vi "Configure AI Filter.vi"(0 "VISA resource name":refnum<visa-resource-name>, 5 "Channel No. (1)":i32=1 min=1 max=6932, 9 "Filter Coefficient(3)":i32=3 min=3 max=300, 11 "error in (no error)":errorcluster) -> (4 "VISA resource name out":refnum<visa-resource-name>, 8 "Channel No.":i32, 15 "error out":errorcluster)   [LabVIEW 2020, in "Yokogawa GX Series.lvlib"]
doc: "Sets the first-order lag filter of the high-speed AI channel.\n\nCommand: SFilter."
uses:
  <instrlib>/Yokogawa GX Series/Yokogawa GX Series.lvlib
panel:
  in  "Use (False)":bool
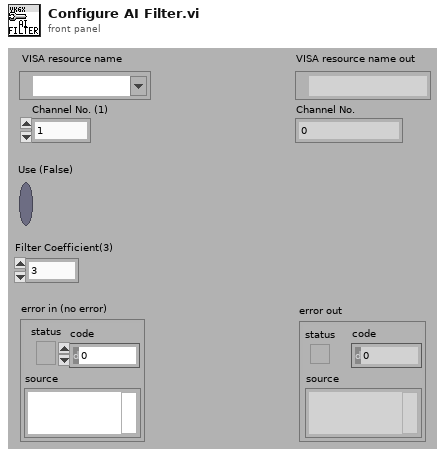
[diagram p1: front panel]
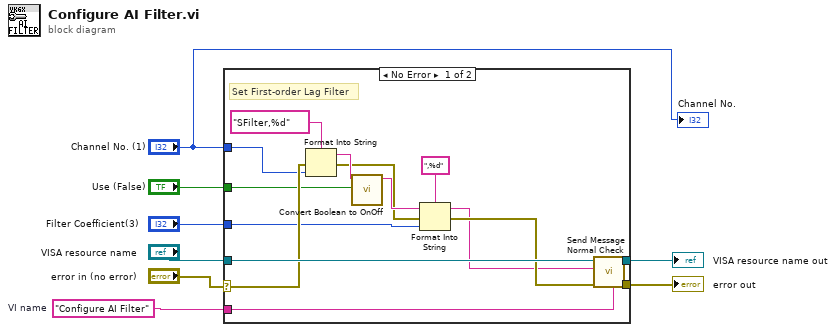
[diagram p0: block diagram]
diagram:
  w4 = "Configure AI Filter"  # VI name
  n1 = case shown="No Error" "error in (no error)" {
    selector: "error in (no error)" -> [w19 w24]
    tunnel: [w23 w25] -> w8
    tunnel: [w22 w24] -> w7
    tunnel: "VISA resource name" -> [w21 w25]
    tunnel: w4 -> [w18 _]
    tunnel: "Channel No. (1)" -> [w17 _]
    tunnel: "Use (False)" -> [w16 _]
    tunnel: "Filter Coefficient(3)" -> [w14 _]
    frame No Error {
      # "Set First-order Lag Filter"
      n2 = Format Into String(format string="SFilter,%d", error in=w19, w17) -> (resulting string=w15:string, error out=w11:errorcluster)  [unwired: 1 in]
      n3 = call <instrlib>:"Convert Boolean to OnOff.vi"("On/Off"=w16, "Initial String (\"\")"=w15) -> ("Resulting String"=w13:string)  [unwired: 9 in]
      n4 = Format Into String(format string=",%d", initial string=w13, error in=w11, w14) -> (resulting string=w9:string, error out=w10:errorcluster)
      n5 = call <instrlib>:"Send Message Normal Check.vi"("Source (\"\")"=w18, "error in (no error)"=w10, "Send Message (\"\")"=w9, "VISA resource name"=w21) -> ("error out"=w22:errorcluster, "VISA resource name out"=w23:refnum<visa-resource-name>)  [unwired: 2 in, 4 out]
    }
    frame Error {
    }
  }
  "error out" <- w7
  "VISA resource name out" <- w8
  "Channel No." <- "Channel No. (1)"
